vi "From JSON Text.vi"   [LabVIEW 2020, in "JSONtext.lvlib"]
doc: "Convert a JSON Value into a LabVIEW data type. Polymorphic; select the type of data. Type may also be specified by a supplied type in a Variant. This may be a cluster of other types."
uses:
  <vilib>/JDP Science/JSONtext/JSONtext.lvlib
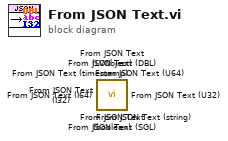
[diagram p0: block diagram]
diagram:
  n1 = call <vilib>:"From JSON Text (boolean).vi"() -> ()  [unwired: 9 in, 3 out]
  n2 = call <vilib>:"From JSON Text (U64).vi"() -> ()  [unwired: 9 in, 3 out]
  n3 = call <vilib>:"From JSON Text (I64).vi"() -> ()  [unwired: 9 in, 3 out]
  n4 = call <vilib>:"From JSON Text (U32).vi"() -> ()  [unwired: 9 in, 3 out]
  n5 = call <vilib>:"From JSON Text (LVObject).vi"() -> ()  [unwired: 9 in, 3 out]
  n6 = call <vilib>:"From JSON Text (timestamp).vi"() -> ()  [unwired: 9 in, 3 out]
  n7 = call <vilib>:"From JSON Text (string).vi"() -> ()  [unwired: 9 in, 3 out]
  n8 = call <vilib>:"From JSON Text (SGL).vi"() -> ()  [unwired: 9 in, 3 out]
  n9 = call <vilib>:"From JSON Text (I32).vi"() -> ()  [unwired: 9 in, 3 out]
  n10 = call <vilib>:"From JSON Text (DBL).vi"() -> ()  [unwired: 9 in, 3 out]
